vi "Class Name.vi"() -> (3 "class name":string)   [LabVIEW 2019, in "DSF Core.lvlib" / "Plugin Interface.lvclass"]
uses:
  Plugin Interface.lvclass
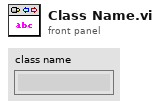
[diagram p1: front panel]
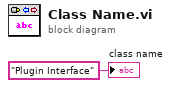
[diagram p0: block diagram]
diagram:
  "class name" <- "Plugin Interface" ("class name")
